vi "FPServerRepository.vi"(0 "reference in":refnum<class "FrontPanelManager.lvclass">, 1 "Action(ReadRepository)":T1(ring), 5 "error in (no error)":errorcluster) -> (9 "ProcessViRef":refnum<vi>, 11 "ProcessSyncQueue":refnum<queue>, 13 "FromProcessQueue":refnum<queue>, 14 "reference out":refnum<class "FrontPanelManager.lvclass">, 15 "ToProcessQueue":refnum<queue>, 17 "ProcessAlreadyStarted":bool, 19 "error out":errorcluster)   [LabVIEW 2014, in "FrontPanelPublisher.lvlib" / "FrontPanelManager.lvclass"]
uses:
  FrontPanelManager.lvclass
  FPServerMessage.ctl
  FPServer.ctl
  FrontPanelManager.lvclass/FrontPanelManager.ctl
  FPServer.vi
panel:
  # "Use this indicator for sending messages to the Process VI"
  # "These indicators are used by the process VIs"
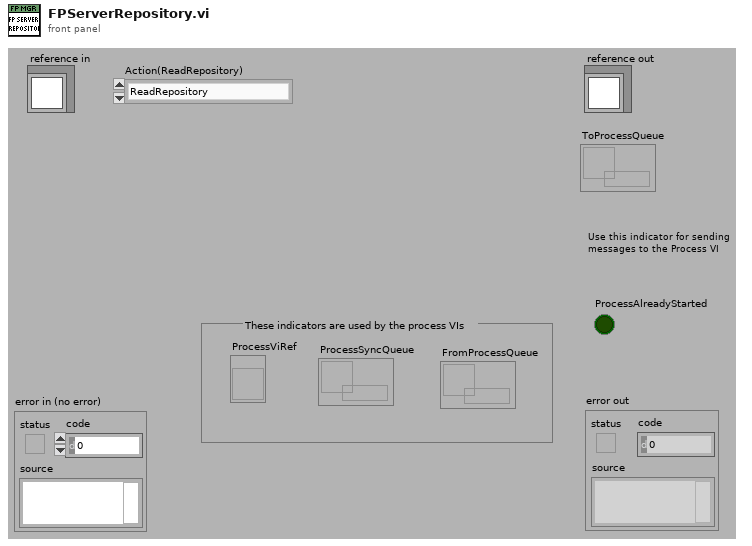
[diagram p1: front panel]
types:
  T1 = enum16{"ReadRepository", "CreateNew", "CreateOrLookUpExisting", "ReadRepositoryAndDestroy"}
  T2 = typedef "FrontPanelPublisher.lvlib/FrontPanelManager.lvclass/FPServer.ctl" = cluster{"ToProcessQueue":refnum<queue>, "FromProcessQueue":refnum<queue>, "ProcessSyncQueue":refnum<queue>, "ProcessViRef":refnum<vi>}
  T3 = typedef "FrontPanelPublisher.lvlib/FrontPanelManager.lvclass/FPServerMessage.ctl" = cluster{"Message":string, "Page":string, "Data":string[][], "Connection ID":u64}
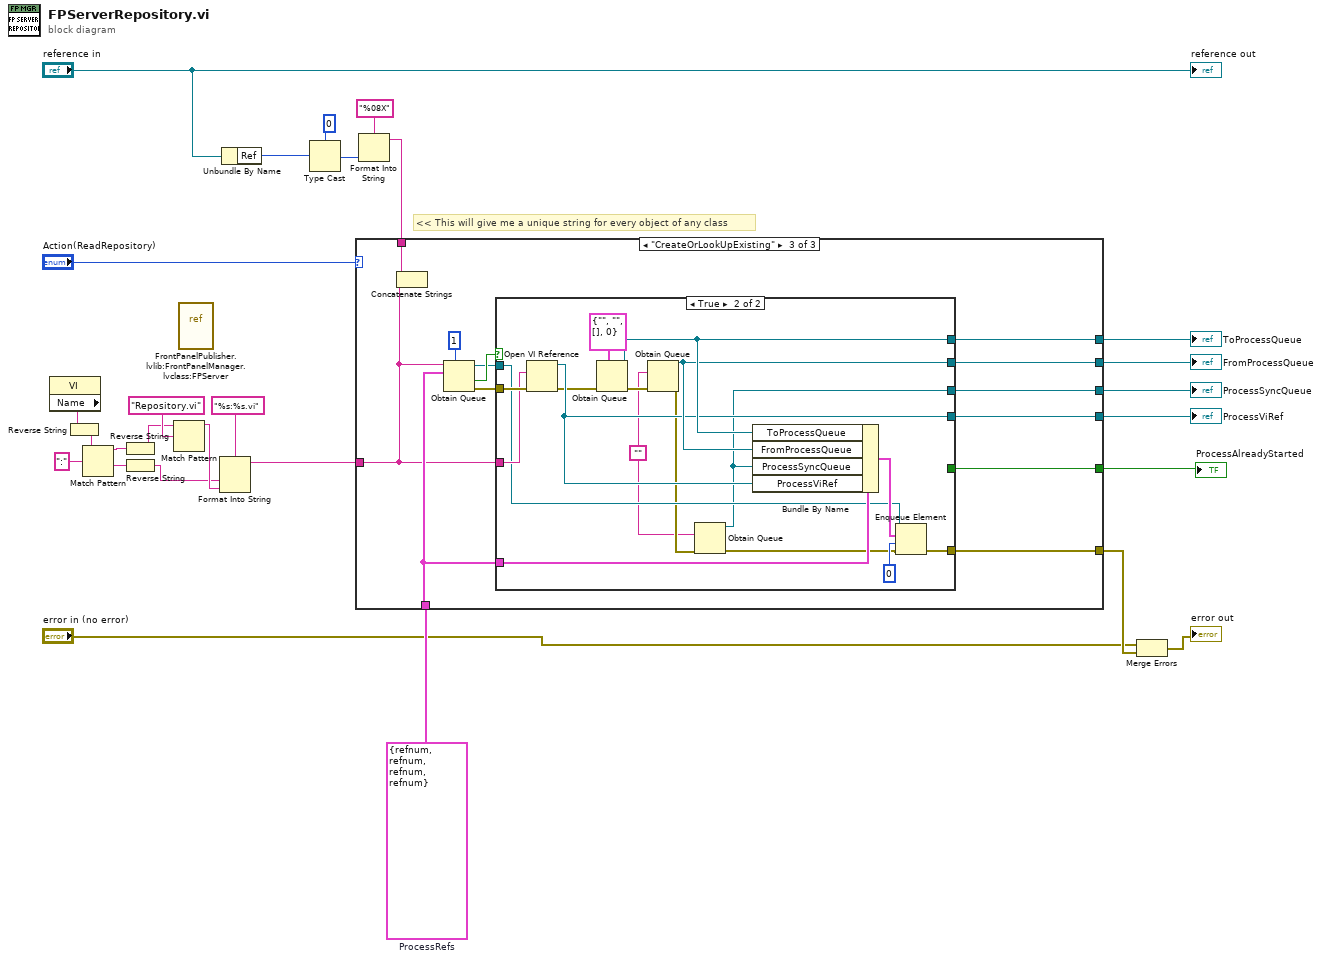
[diagram p0: block diagram]
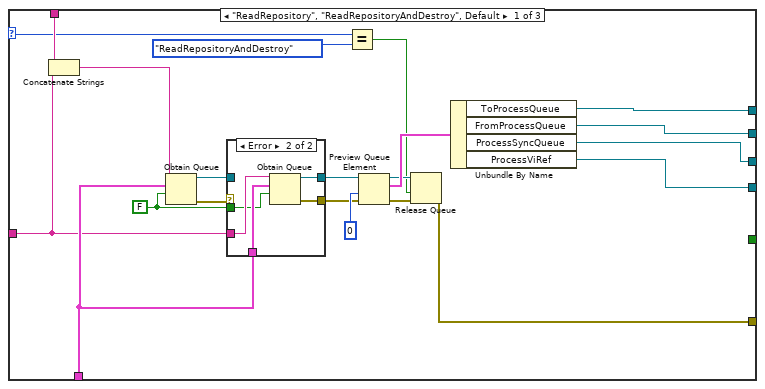
[diagram p2: hidden frame]
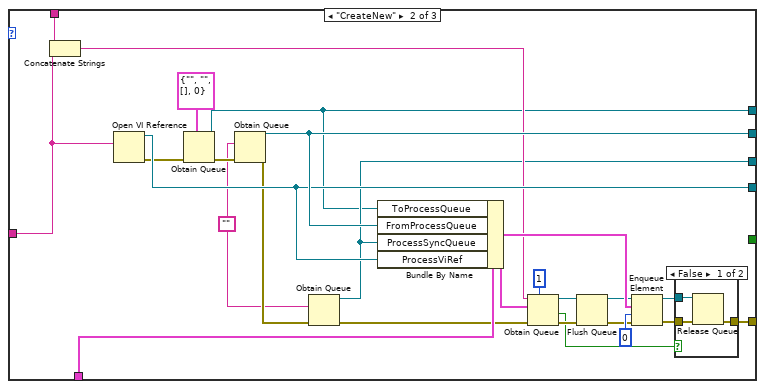
[diagram p4: hidden frame]
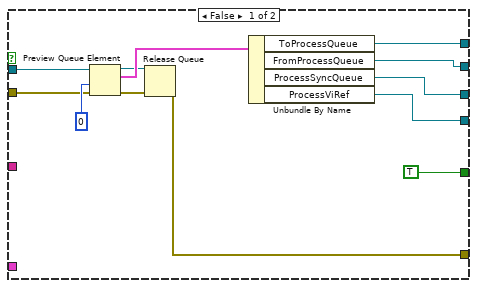
[diagram p6: hidden frame]
diagram:
  w22 = T2 {"ToProcessQueue"=refnum, "FromProcessQueue"=refnum, "ProcessSyncQueue"=refnum, "ProcessViRef"=refnum}  # ProcessRefs
  # "<< This will give me a unique string for every object of any class"
  n1 = property class="VI"() -> ("Name"=w11:string)  [unwired: 2 in, 2 out]
  n2 = Reverse String(1:w11) -> (0:w12:string)
  n3 = Match Pattern(string=w12, regular expression=":") -> (before substring=w16:string, after substring=w13:string)  [unwired: 1 in, 2 out]
  n4 = Reverse String(1:w16) -> (0:w17:string)
  n5 = Reverse String(1:w13) -> (0:w15:string)
  n6 = Match Pattern(string=w17, regular expression="Repository.vi") -> (before substring=w19:string)  [unwired: 1 in, 3 out]
  n7 = vi-ref "FrontPanelPublisher.lvlib:FrontPanelManager.lvclass:FPServer.vi"() -> ()  [unwired: 1 out]
  n8 = Format Into String(format string="%s:%s.vi", w15, w19) -> (resulting string=w9:string)  [unwired: 2 in, 1 out]
  n9 = Unbundle By Name("reference in") -> ("Ref"=w1:u32)
  n10 = Type Cast(type=u32 0, x=w1) -> (*(type *) &x=w6:u32)
  n11 = Format Into String(format string="%08X", w6) -> (resulting string=w3:string)  [unwired: 2 in, 1 out]
  n12 = case shown="\"CreateOrLookUpExisting\"" "Action(ReadRepository)" {
    selector: "Action(ReadRepository)" -> [w29 _ _]
    tunnel: [w43 w66 w95] -> w26
    tunnel: [w45 w56 w97] -> w24
    tunnel: [w44 w80 w96] -> w25
    tunnel: [w46 w79 w94] -> w23
    tunnel: w22 -> [w38 w72 w90]
    tunnel: w3 -> [w36 w71 w86]
    tunnel: [w31 w59 w93] -> w20
    tunnel: w9 -> [w35 w69 w85]
    tunnel: [_ _ w88] -> w8
    frame "ReadRepository", "ReadRepositoryAndDestroy", Default {
      w37 = FALSE ("create if not found? (T)")
      n13 = Concatenate Strings(w36, w35) -> (w34:string)
      n14 = Obtain Queue(name (unnamed)=w34, element data type=w38, create if not found? (T)=w37) -> (queue out=w40:refnum<queue>, error out=w42:errorcluster)  [unwired: 2 in, 1 out]
      n15 = case shown="Error" w42 {
        selector: w42 -> [w50 _]
        tunnel: [w50 w52] -> w41
        tunnel: w40 -> [w49 _]
        tunnel: [w49 w53] -> w39
        tunnel: w38 -> [_ w55]
        tunnel: w35 -> [_ w54]
        tunnel: w37 -> [_ w51]
        frame No Error {
        }
        frame Error {
          n16 = Obtain Queue(name (unnamed)=w54, element data type=w55, create if not found? (T)=w51) -> (queue out=w53:refnum<queue>, error out=w52:errorcluster)  [unwired: 2 in, 1 out]
        }
      }
      n17 = Equal?(x=w29, y=T1."ReadRepositoryAndDestroy") -> (x = y?=w28:bool)
      n18 = Preview Queue Element(queue=w39, timeout in ms (-1)=0, error in (no error)=w41) -> (queue out=w33:refnum<queue>, element=w47:T2, error out=w32:errorcluster)  [unwired: 1 out]
      n19 = Release Queue(queue=w33, force destroy? (F)=w28, error in (no error)=w32) -> (error out=w31:errorcluster)  [unwired: 2 out]
      n20 = Unbundle By Name(w47) -> ("ToProcessQueue"=w45:refnum<queue>, "FromProcessQueue"=w44:refnum<queue>, "ProcessSyncQueue"=w43:refnum<queue>, "ProcessViRef"=w46:refnum<vi>)
    }
    frame "CreateNew" {
      w65 = ""
      n21 = Concatenate Strings(w71, w69) -> (w70:string)
      n22 = Open VI Reference(vi path=w69) -> (vi reference=w79:refnum<vi>, error out=w77:errorcluster)  [unwired: 5 in]
      n23 = Obtain Queue(element data type=T3 {"Message"="", "Page"="", "Data"=[], "Connection ID"=0} ("Process Message"), error in (no error)=w77) -> (queue out=w56:refnum<queue>, error out=w78:errorcluster)  [unwired: 3 in, 1 out]
      n24 = Obtain Queue(element data type=w65, error in (no error)=w78) -> (queue out=w80:refnum<queue>, error out=w68:errorcluster)  [unwired: 3 in, 1 out]
      n25 = Obtain Queue(element data type=w65, error in (no error)=w68) -> (queue out=w66:refnum<queue>, error out=w67:errorcluster)  [unwired: 3 in, 1 out]
      n26 = Bundle By Name(cluster=w72, "ToProcessQueue"=w56, "FromProcessQueue"=w80, "ProcessSyncQueue"=w66, "ProcessViRef"=w79) -> (w75:T2)
      n27 = Obtain Queue(max queue size (-1, unlimited)=1, name (unnamed)=w70, element data type=w75, error in (no error)=w67) -> (queue out=w76:refnum<queue>, created new?=w58:bool, error out=w63:errorcluster)  [unwired: 1 in]
      n28 = Flush Queue(queue=w76, error in (no error)=w63) -> (queue out=w64:refnum<queue>, error out=w62:errorcluster)  [unwired: 1 out]
      n29 = Enqueue Element(queue=w64, element=w75, timeout in ms (-1)=0, error in (no error)=w62) -> (queue out=w61:refnum<queue>, error out=w60:errorcluster)  [unwired: 1 out]
      n30 = case shown="False" w58 {
        tunnel: w60 -> [w83 w84]
        tunnel: w61 -> [w82 _]
        tunnel: [w81 w84] -> w59
        frame False {
          n31 = Release Queue(queue=w82, error in (no error)=w83) -> (error out=w81:errorcluster)  [unwired: 1 in, 2 out]
        }
        frame True {
        }
      }
    }
    frame "CreateOrLookUpExisting" {
      n32 = Concatenate Strings(w86, w85) -> ()  [unwired: 1 out]
      n33 = Obtain Queue(max queue size (-1, unlimited)=1, name (unnamed)=w85, element data type=w90) -> (queue out=w91:refnum<queue>, created new?=w92:bool, error out=w89:errorcluster)  [unwired: 2 in]
      n34 = case shown="True" w92 {
        tunnel: [w109 w126] -> w97
        tunnel: [w108 w125] -> w96
        tunnel: [w107 w111] -> w95
        tunnel: [w106 w124] -> w94
        tunnel: [w98 w123] -> w93
        tunnel: w90 -> [_ w122]
        tunnel: w89 -> [w103 w117]
        tunnel: w85 -> [_ w116]
        tunnel: w91 -> [w104 w115]
        tunnel: [TRUE _] -> w88
        frame False {
          n35 = Preview Queue Element(queue=w104, timeout in ms (-1)=0, error in (no error)=w103) -> (queue out=w100:refnum<queue>, element=w102:T2, error out=w99:errorcluster)  [unwired: 1 out]
          n36 = Release Queue(queue=w100, error in (no error)=w99) -> (error out=w98:errorcluster)  [unwired: 1 in, 2 out]
          n37 = Unbundle By Name(w102) -> ("ToProcessQueue"=w109:refnum<queue>, "FromProcessQueue"=w108:refnum<queue>, "ProcessSyncQueue"=w107:refnum<queue>, "ProcessViRef"=w106:refnum<vi>)
        }
        frame True {
          w112 = ""
          n38 = Open VI Reference(vi path=w116, error in (no error)=w117) -> (vi reference=w124:refnum<vi>, error out=w120:errorcluster)  [unwired: 4 in]
          n39 = Obtain Queue(element data type=T3 {"Message"="", "Page"="", "Data"=[], "Connection ID"=0} ("Process Message"), error in (no error)=w120) -> (queue out=w126:refnum<queue>, error out=w121:errorcluster)  [unwired: 3 in, 1 out]
          n40 = Obtain Queue(element data type=w112, error in (no error)=w121) -> (queue out=w125:refnum<queue>, error out=w114:errorcluster)  [unwired: 3 in, 1 out]
          n41 = Obtain Queue(element data type=w112, error in (no error)=w114) -> (queue out=w111:refnum<queue>, error out=w113:errorcluster)  [unwired: 3 in, 1 out]
          n42 = Bundle By Name(cluster=w122, "ToProcessQueue"=w126, "FromProcessQueue"=w125, "ProcessSyncQueue"=w111, "ProcessViRef"=w124) -> (w119:T2)
          n43 = Enqueue Element(queue=w115, element=w119, timeout in ms (-1)=0, error in (no error)=w113) -> (error out=w123:errorcluster)  [unwired: 2 out]
        }
      }
    }
  }
  "ProcessSyncQueue" <- w26
  "ToProcessQueue" <- w24
  "FromProcessQueue" <- w25
  "ProcessViRef" <- w23
  "ProcessAlreadyStarted" <- w8
  n44 = Merge Errors("error in (no error)", w20) -> (→"error out":errorcluster)
  "reference out" <- "reference in"
